vi "SIM_Drive_INIT.vi"(8 "error in (no error)":errorcluster, 9 "Module Positions":T1[](array[typedef]) {"Angle"."SIN" format="%13.4f"; "Angle"."COS" format="%13.4f"; "Angle"."VALUE" format="%13.4f"}, 10 "Simulation_Kinematics":T3 {"SavedModuleStates"."Angle"."SIN" format="%13.4f"; "SavedModuleStates"."Angle"."COS" format="%13.4f"; "SavedModuleStates"."Angle"."VALUE" format="%13.4f"; "PrevCoR"."Y" format="%14.3f"; "PrevCoR"."X" format="%14.3f"; "Modules"."Y" format="%14.3f"; "Modules"."X" format="%14.3f"}, 11 "Initial Robot Position":T7 {"ROTATION"."SIN" format="%13.4f"; "ROTATION"."COS" format="%13.4f"; "ROTATION"."VALUE" format="%13.4f"; "TRANSLATION"."Y" format="%14.3f"; "TRANSLATION"."X" format="%14.3f"}) -> (0 "error out":errorcluster)   [LabVIEW 2023]
uses:
  <vilib>/Rock Robotics/WPI/ThirdParty/JAS_Junk/TrajLib/TypeDef/POSE2D.ctl
  <vilib>/Rock Robotics/WPI/ThirdParty/JAS_Junk/TrajLib/TypeDef/TRANSLATION2D.ctl
  <vilib>/Rock Robotics/WPI/ThirdParty/JAS_Junk/TrajLib/TypeDef/ROTATION2D.ctl
  <vilib>/Rock Robotics/WPI/ThirdParty/JAS_Junk/TrajLib/TypeDef/SWERVE_DRIVE_KINEMATICS.ctl
  <vilib>/Analysis/Matrix/Datatypes/RealMatrix.ctl
  <vilib>/Rock Robotics/WPI/ThirdParty/JAS_Junk/TrajLib/TypeDef/SWERVE_DRIVE_MODULE_STATE.ctl
  <vilib>/Rock Robotics/WPI/ThirdParty/JAS_Junk/TrajLib/TypeDef/SWERVE_DRIVE_MODULE_POSITION.ctl
  <vilib>/Rock Robotics/SystemInterfaces/DIO/FPGA_DIOPWMChannel.ctl
  <vilib>/Rock Robotics/SystemInterfaces/DIO/FPGA_DIOChannel.ctl
  <vilib>/Rock Robotics/WPI/ThirdParty/JAS_Junk/TrajLib/Conv_Deg_Radians.vi
  <vilib>/Rock Robotics/WPI/ThirdParty/JAS_Junk/TrajLib/Rotation2d_CreateAngle.vi
  SIM_Drive_Globals.vi
  <vilib>/Rock Robotics/WPI/ThirdParty/JAS_Junk/TrajLib/Trajectory_Library.lvlib
  <vilib>/Analysis/Matrix/NI_Matrix.lvlib
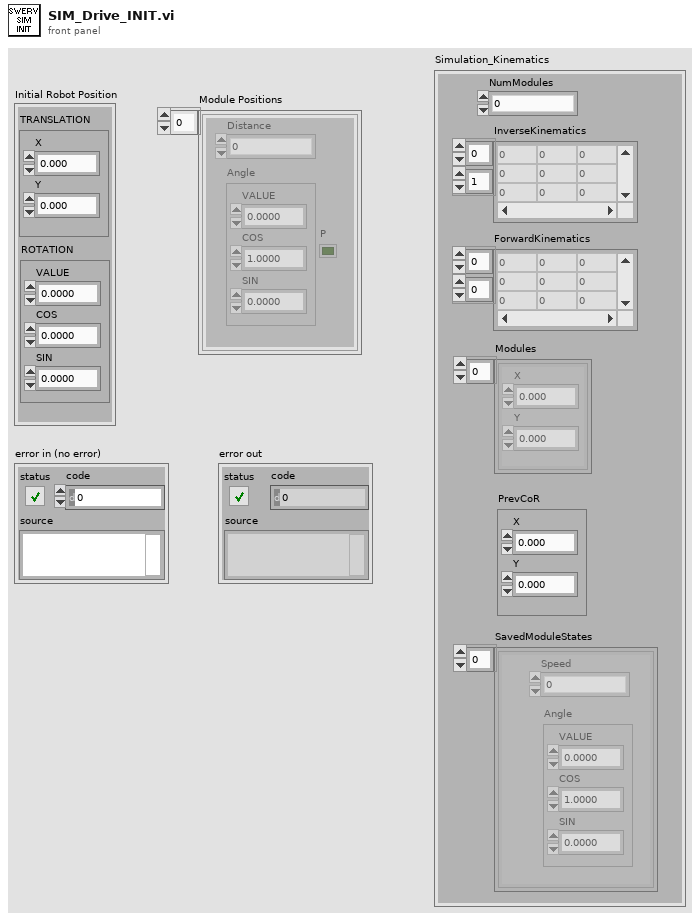
[diagram p1: front panel]
types:
  T1 = typedef "Trajectory_Library.lvlib/SWERVE_DRIVE_MODULE_POSITION.ctl" = cluster{"Distance":dbl, "Angle":T2, "P":bool}
  T2 = typedef "Trajectory_Library.lvlib/ROTATION2D.ctl" = cluster{"VALUE":dbl, "COS":dbl, "SIN":dbl}
  T3 = typedef "Trajectory_Library.lvlib/SWERVE_DRIVE_KINEMATICS.ctl" = cluster{"NumModules":i32, "InverseKinematics":T4, "ForwardKinematics":T4, "Modules":T5[], "PrevCoR":T5, "SavedModuleStates":T6[]}
  T4 = typedef "NI_Matrix.lvlib/RealMatrix.ctl" = dbl[][]
  T5 = typedef "Trajectory_Library.lvlib/TRANSLATION2D.ctl" = cluster{"X":dbl, "Y":dbl}
  T6 = typedef "Trajectory_Library.lvlib/SWERVE_DRIVE_MODULE_STATE.ctl" = cluster{"Speed":dbl, "Angle":T2}
  T7 = typedef "Trajectory_Library.lvlib/POSE2D.ctl" = cluster{"TRANSLATION":T5, "ROTATION":T2}
  T8 = typedef "FPGA_DIOChannel.ctl" = enum8{"DIO 0", "DIO 1", "DIO 2", "DIO 3", "DIO 4", "DIO 5", "DIO 6", "DIO 7", "DIO 8", "DIO 9", "DIO MXP 0", "DIO MXP 1", "DIO MXP 2", "DIO MXP 3", "DIO MXP 4", "DIO MXP 5", "DIO MXP 6", "DIO MXP 7", "DIO MXP 8", "DIO MXP 9", "DIO MXP 10", "DIO MXP 11", "DIO MXP 12", "DIO MXP 13", "DIO MXP 14", "DIO MXP 15", "SPI Port CS1", "SPI Port CS2", "SPI Port CS3", "SPI Port MISO", "SPI Port MOSI", "Invalid"}
  T9 = typedef "FPGA_DIOPWMChannel.ctl" = enum8{"PWM 0", "PWM 1", "PWM 2", "PWM 3", "PWM 4", "PWM 5", "PWM 6", "PWM 7", "PWM 8", "PWM 9", "PWM MXP 0", "PWM MXP 1", "PWM MXP 2", "PWM MXP 3", "PWM MXP 4", "PWM MXP 5", "PWM MXP 6", "PWM MXP 7", "PWM MXP 8", "PWM MXP 9", "Invalid"}
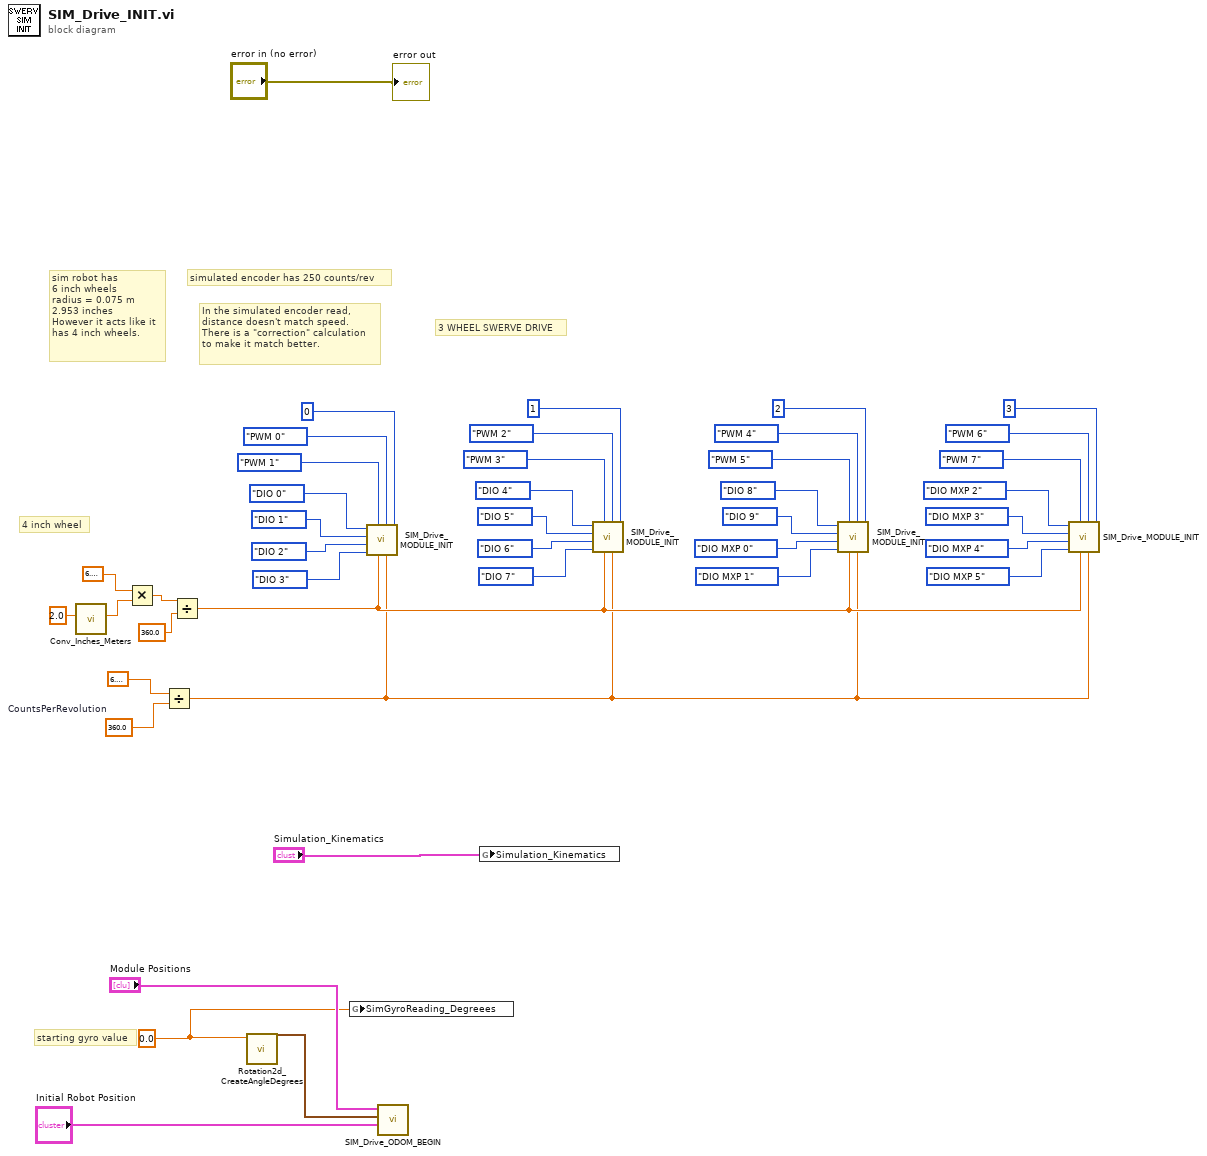
[diagram p0: block diagram]
diagram:
  w1 = 0.0
  w18 = 360.0  # CountsPerRevolution
  # "starting gyro value"
  # "4 inch wheel"
  # "3 WHEEL SWERVE DRIVE"
  # "In the simulated encoder read,\ndistance doesn't match speed.\nThere is a \"correction\" calculation\nto make it match better."
  # "simulated encoder has 250 counts/rev"
  # "sim robot has\n6 inch wheels\nradius = 0.075 m\n2.953 inches\nHowever it acts like it\nhas 4 inch wheels."
  n1 = call <vilib>:"Conv_Inches_Meters.vi"("INCH"=2.0) -> ("Meters"=w33:dbl)  [unwired: 10 in]
  n2 = Multiply(x=6.283185307179586, y=w33) -> (x*y=w7:dbl)
  n3 = Divide(x=6.283185307179586, y=w18) -> (x/y=w42:dbl)
  n4 = Divide(x=w7, y=360.0) -> (x/y=w43:dbl)
  n5 = call <vilib>:"Rotation2d_CreateAngleDegrees.vi"("Angle_Degrees"=w1) -> ("ROTATION"=w4:T2)  [unwired: 10 in]
  n6 = global write "SIM_Drive_Globals.vi" "SimGyroReading_Degreees"(w1) -> ()
  n7 = call "SIM_Drive_MODULE_INIT.vi"("Module Index"=0 ("NameSuffix"), "SwerveRadiansPerCount"=w42, "Drive PWM Channel"=FPGA_DIOPWMChannel."PWM 0", "DriveDistPerCount"=w43, "Swerve PWM Channel"=FPGA_DIOPWMChannel."PWM 1", "Swerve B Channel"=FPGA_DIOChannel."DIO 3", "Swerver A Channel"=FPGA_DIOChannel."DIO 2", "Drive B Channel"=FPGA_DIOChannel."DIO 1", "Drive A channel"=FPGA_DIOChannel."DIO 0") -> ()  [unwired: 3 in]
  n8 = call "SIM_Drive_ODOM_BEGIN.vi"("Initial Pose"="Initial Robot Position", "Initial Gyro Angle"=w4, "Module Positions"="Module Positions") -> ()  [unwired: 8 in, 1 out]
  n9 = global write "SIM_Drive_Globals.vi" "Simulation_Kinematics"("Simulation_Kinematics") -> ()
  n10 = call "SIM_Drive_MODULE_INIT.vi"("Module Index"=1 ("NameSuffix"), "SwerveRadiansPerCount"=w42, "Drive PWM Channel"=FPGA_DIOPWMChannel."PWM 2", "DriveDistPerCount"=w43, "Swerve PWM Channel"=FPGA_DIOPWMChannel."PWM 3", "Swerve B Channel"=FPGA_DIOChannel."DIO 7", "Swerver A Channel"=FPGA_DIOChannel."DIO 6", "Drive B Channel"=FPGA_DIOChannel."DIO 5", "Drive A channel"=FPGA_DIOChannel."DIO 4") -> ()  [unwired: 3 in]
  n11 = call "SIM_Drive_MODULE_INIT.vi"("Module Index"=2 ("NameSuffix"), "SwerveRadiansPerCount"=w42, "Drive PWM Channel"=FPGA_DIOPWMChannel."PWM 4", "DriveDistPerCount"=w43, "Swerve PWM Channel"=FPGA_DIOPWMChannel."PWM 5", "Swerve B Channel"=FPGA_DIOChannel."DIO MXP 1", "Swerver A Channel"=FPGA_DIOChannel."DIO MXP 0", "Drive B Channel"=FPGA_DIOChannel."DIO 9", "Drive A channel"=FPGA_DIOChannel."DIO 8") -> ()  [unwired: 3 in]
  n12 = call "SIM_Drive_MODULE_INIT.vi"("Module Index"=3 ("NameSuffix"), "SwerveRadiansPerCount"=w42, "Drive PWM Channel"=FPGA_DIOPWMChannel."PWM 6", "DriveDistPerCount"=w43, "Swerve PWM Channel"=FPGA_DIOPWMChannel."PWM 7", "Swerve B Channel"=FPGA_DIOChannel."DIO MXP 5", "Swerver A Channel"=FPGA_DIOChannel."DIO MXP 4", "Drive B Channel"=FPGA_DIOChannel."DIO MXP 3", "Drive A channel"=FPGA_DIOChannel."DIO MXP 2") -> ()  [unwired: 3 in]
  "error out" <- "error in (no error)"
